vi "AssetInterface_Update Tags_Wrapper_deleteme.vi"(8 "error in (no error)":errorcluster, 10 "data value reference":refnum<data-value>, 11 "Asset_Interface in":refnum<class "AssetInterface.lvclass">) -> (0 "error out":errorcluster, 3 "Asset_Interface out":refnum<class "AssetInterface.lvclass">)   [LabVIEW 2015]
uses:
  AssetInterface.lvclass
  System/System.lvclass
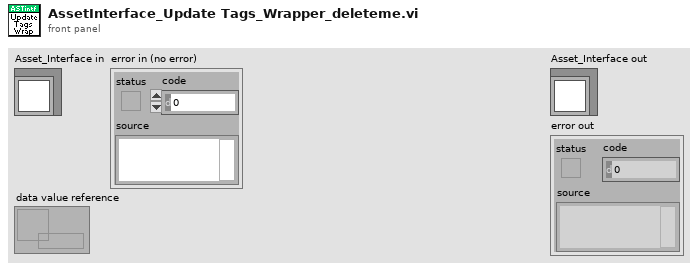
[diagram p1: front panel]
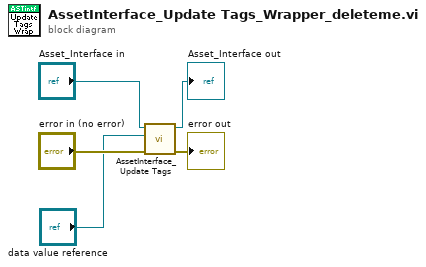
[diagram p0: block diagram]
diagram:
  n1 = call-dynamic "AssetInterface_Update Tags.vi"("error in (no error)"="error in (no error)", "TagBus DVR"="data value reference", "Asset_Interface in"="Asset_Interface in") -> ("error out"=→"error out":errorcluster, "Asset_Interface out"=→"Asset_Interface out":refnum<class "AssetInterface.lvclass">)  [unwired: 6 in, 1 out]
